vi "Introduce.vi"(8 "Error In":errorcluster, 11 "Droid in":refnum<class "Droid.lvclass">) -> (0 "Error Out":errorcluster, 3 "Droid out":refnum<class "Droid.lvclass">)   [LabVIEW 2021, in "Droid.lvclass"]
doc: "Show ID of droid in prompt message for user. Comments in Polish."
uses:
  Droid.lvclass
  Droid.lvclass/Droid.ctl
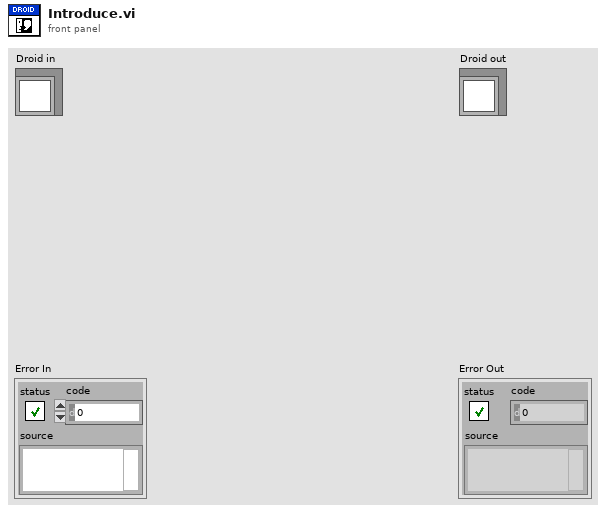
[diagram p1: front panel]
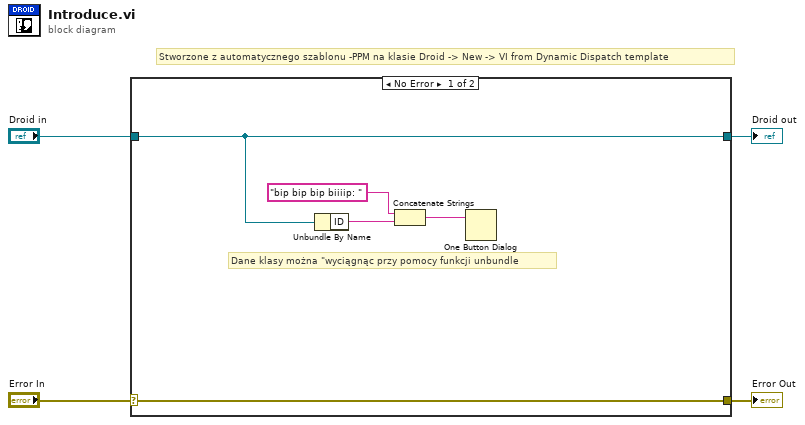
[diagram p0: block diagram]
diagram:
  # "Stworzone z automatycznego szablonu -PPM na klasie Droid -> New -> VI from Dynamic Dispatch template"
  n1 = case shown="No Error" "Error In" {
    selector: "Error In" -> [w9 w11]
    tunnel: [w9 w11] -> w3
    tunnel: [w8 w10] -> w1
    tunnel: "Droid in" -> [w8 w10]
    frame No Error {
      # "Dane klasy można \"wyciągnąc przy pomocy funkcji unbundle"
      n2 = Unbundle By Name(w8) -> ("ID"=w7:string)
      n3 = Concatenate Strings("bip bip bip biiiip: ", w7) -> (w5:string)
      n4 = One Button Dialog(message=w5) -> ()  [unwired: 1 in, 1 out]
    }
    frame Error {
    }
  }
  "Error Out" <- w3
  "Droid out" <- w1
